vi "WFGetDtFs.vi"(11 "Waveform":waveform(dbl)={"t0"=timestamp(0 s since 1904-01-01), "dt"=0.0, "Y"=[]}) -> (0 "Fs (Hz)":dbl, 3 "dt":dbl)   [LabVIEW 2013]
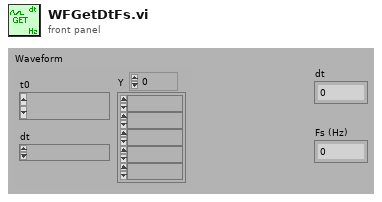
[diagram p1: front panel]
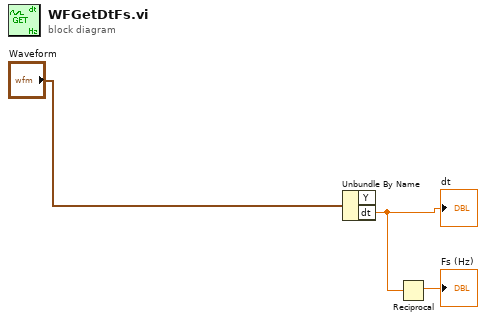
[diagram p0: block diagram]
diagram:
  n1 = Unbundle By Name("Waveform") -> ("dt"=w1:dbl)  [unwired: 1 out]
  "dt" <- w1
  n2 = Reciprocal(x=w1) -> (1/x=→"Fs (Hz)":dbl)
